vi "Frame.vi"(8 "error in (no error)":errorcluster, 11 "Node Ptr":T1 format="%.0x") -> (0 "error out":errorcluster)   [LabVIEW 2015, in "Diagnostics Addon System Explorer.lvlib"]
uses:
  Diagnostics Addon System Explorer.lvlib
  <vilib>/NI Veristand/Custom Device API/Custom Device Item Ref.ctl
  Shared/FG Action.ctl
  Shared/Signal Parameters FG.vi
  Shared/GUID Lookup.vi
  <vilib>/NI Veristand/Custom Device API/NI VeriStand - Set Item Property.vi
  <vilib>/NI Veristand/Custom Device API/Set Item Property (U32).vi
  <vilib>/NI Veristand/Custom Device API/NI VeriStand - Get Item Property.vi
  <vilib>/NI Veristand/Custom Device API/Get Item Property (U32).vi
  <vilib>/NI Veristand/Custom Device API/NI VeriStand - Get Item Children.vi
  <vilib>/NI Veristand/Custom Device API/Set Item Property (Double).vi
  <vilib>/NI Veristand/Custom Device API/Set Item Property (String).vi
  <vilib>/NI Veristand/Custom Device API/Get Item Property (Double).vi
  <vilib>/NI Veristand/Custom Device API/Get Item Property (String).vi
  <vilib>/NI Veristand/Custom Device API/NI VeriStand - Get Custom Device Channel Data.vi
  <vilib>/NI Veristand/Custom Device API/Custom Device API.lvlib
  Shared/Diagnostics Addon Shared.lvlib
panel:
  out "Length":u32 caption="Length (bytes)"
  in  "ID":u16 format="%.0x"
  out "Signals":i32(listbox)
  in  "Description":string
  in  "Name":string
  in  "SHDocVw.IWebBrowser":refnum<k7>(container)
  in  "Header":cluster{"Section Name":string}={"Section Name"="Custom Device Item Settings"}
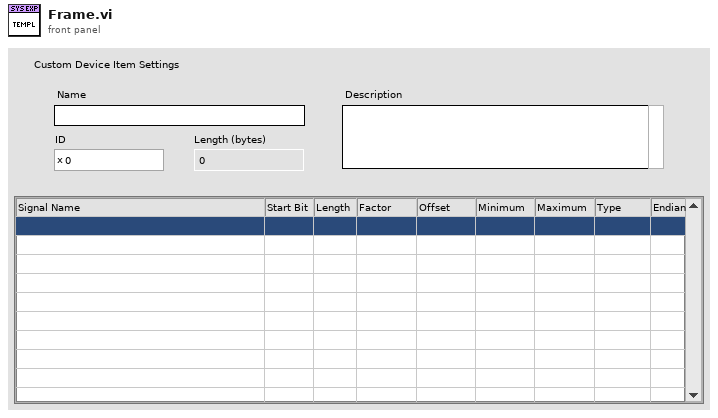
[diagram p1: front panel]
types:
  T1 = typedef "Custom Device API.lvlib/Custom Device Item Ref.ctl" = u64
  T2 = typedef "Diagnostics Addon System Explorer.lvlib/FG Action.ctl" = enum16{"Get", "Set"}
  T3 = typedef "Custom Device API.lvlib/Custom Device Item Info.ctl" = cluster{"Name":string, "Is Channel":bool, "GUID":string, "Is Waveform":bool}
  T4 = typedef "Diagnostics Addon Shared.lvlib/Signal Parameters.ctl" = cluster{"Start Bit":u8, "Length":u8, "Scaling Factor":dbl, "Scaling Offset":dbl, "Minimum":dbl, "Maximum":dbl, "Data Type":u32, "Byte Order":u32, "Default Value":dbl, "Name":string, "Units":string, "Description":string}
  T5 = typedef "Custom Device API.lvlib/Custom Device Commands.ctl" = enum16{"Default", "Item renamed", "Shutdown", "Dynamic button pressed"}
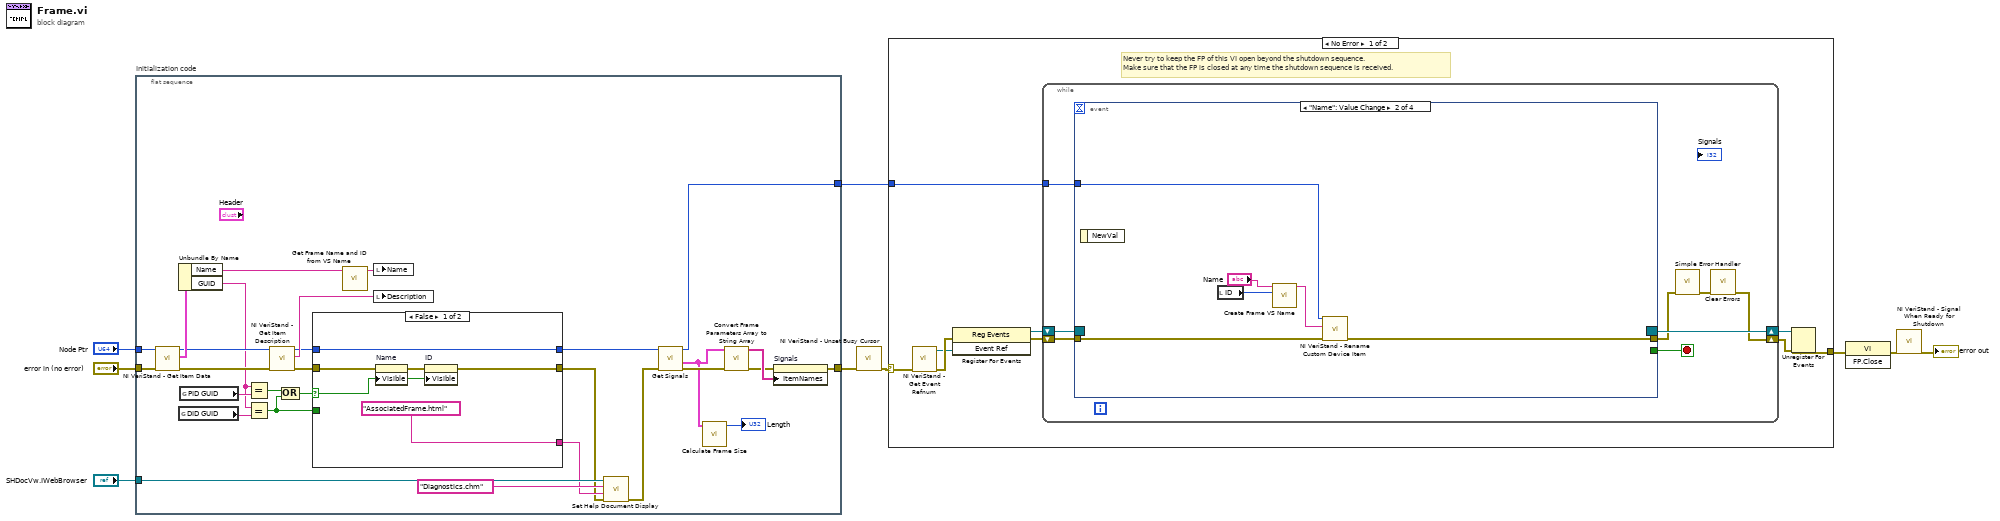
[diagram p0: block diagram]
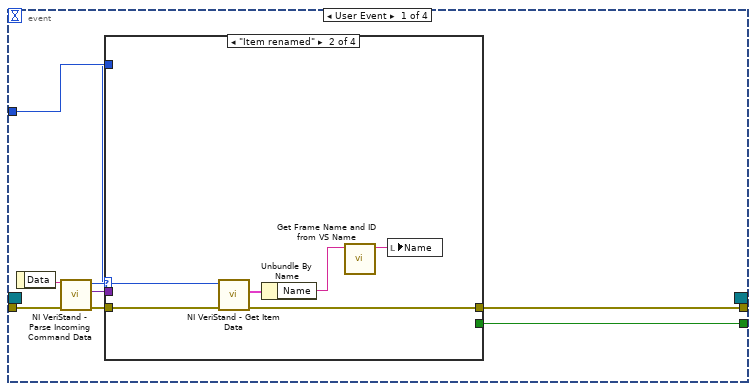
[diagram p2: hidden frame]
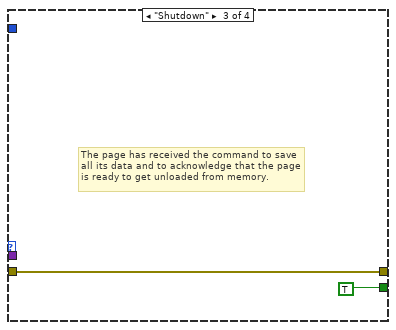
[diagram p4: hidden frame]
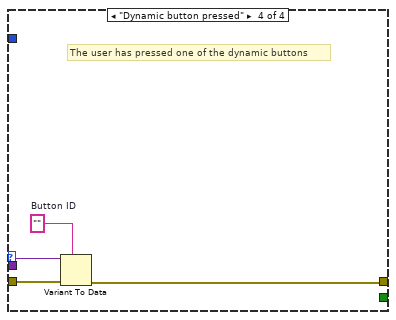
[diagram p5: hidden frame]
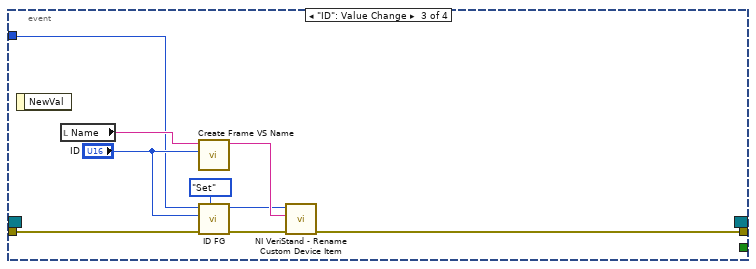
[diagram p6: hidden frame]
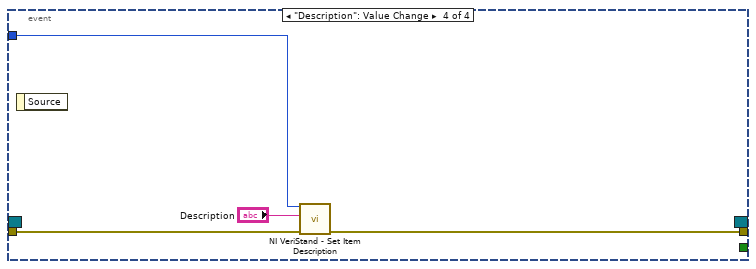
[diagram p7: hidden frame]
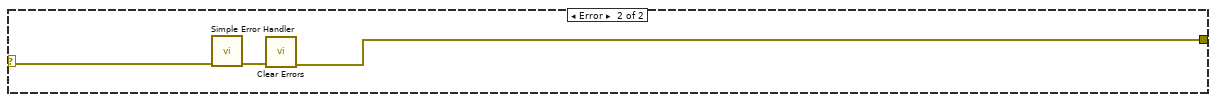
[diagram p8: hidden frame]
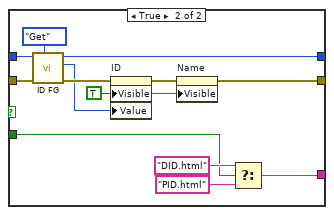
[diagram p9: hidden frame]
diagram:
  n1 = flat-sequence "Initialization code" {
    tunnel: "error in (no error)" -> [w21]
    tunnel: "Node Ptr" -> [w20]
    tunnel: [w33] -> w5
    tunnel: [w36] -> w2
    tunnel: "SHDocVw.IWebBrowser" -> [w19]
    frame #0 {
      n2 = call <vilib>:"NI VeriStand - Get Item Data.vi"("error in (no error)"=w21, "Item Ref in"=w20) -> ("error out"=w22:errorcluster, "Item Info"=w37:T3, "Item Ref out"=w23:T1)  [unwired: 7 out]
      n3 = Unbundle By Name(w37) -> ("Name"=w29:string, "GUID"=w13:string)
      n4 = global read "GUID Lookup.vi" "DID GUID"() -> (w15:string)
      n5 = global read "GUID Lookup.vi" "PID GUID"() -> (w25:string)
      n6 = Equal?(x=w13, y=w25) -> (x = y?=w24:bool)
      n7 = Equal?(x=w13, y=w15) -> (x = y?=w12:bool)
      n8 = call <vilib>:"NI VeriStand - Get Item Description.vi"("error in (no error)"=w22, "Item Ref in"=w23) -> ("error out"=w27:errorcluster, "Description"=w38:string, "Item Ref out"=w26:T1)  [unwired: 7 out]
      n9 = Compound Arithmetic op=OR(w24, w12) -> (w14:bool)
      n10 = case shown="False" w14 {
        selector: w14 -> [w41 _]
        tunnel: [w43 w50] -> w17
        tunnel: [w40 w57] -> w34
        tunnel: w27 -> [w42 w55]
        tunnel: w26 -> [w40 w54]
        tunnel: ["AssociatedFrame.html" ("HTML File") w47] -> w18
        tunnel: w12 -> [_ w45]
        frame False {
          n11 = property on="Name" class="Str"(error in=w42, "Visible"=w41) -> (error out=w44:errorcluster)  [unwired: 1 in, 1 out]
          n12 = property on="ID" class="DigNum (strict)"(error in=w44, "Visible"=w41) -> (error out=w43:errorcluster)  [unwired: 1 in, 1 out]
        }
        frame True {
          w49 = TRUE ("Visible")
          n13 = call "ID FG.vi"("Action"=FG_Action."Get", "error in (no error)"=w55, "Device Item Ref in"=w54) -> ("error out"=w53:errorcluster, "ID"=w52:u32, "Device Item Ref out"=w57:T1)  [unwired: 6 in]
          n14 = property on="ID" class="DigNum (strict)"(error in=w53, "Visible"=w49, "Value"=w52) -> (error out=w51:errorcluster)  [unwired: 1 in, 1 out]
          n15 = property on="Name" class="Str"(error in=w51, "Visible"=w49) -> (error out=w50:errorcluster)  [unwired: 1 in, 1 out]
          n16 = Select(t="DID.html" ("HTML File"), s=w45, f="PID.html" ("HTML File")) -> (s? t:f=w47:string)
        }
      }
      n17 = call "Get Frame Name and ID from VS Name.vi"("VS PID Name"=w29) -> ("PID Name"=w28:string)  [unwired: 9 in, 1 out]
      n18 = local write "Name"(w28) -> ()
      n19 = local write "Description"(w38) -> ()
      n20 = call "Set Help Document Display.vi"("error in (no error)"=w17, "HTML File"=w18, "Main CHM File"="Diagnostics.chm", "SHDocVw.IWebBrowser2"=w19) -> ("error out"=w16:errorcluster)  [unwired: 7 in]
      n21 = call "Get Signals.vi"("error in (no error)"=w16, "Device Item Ref out"=w34) -> ("error out"=w31:errorcluster, "Parameters"=w11:T4[], "Item Ref out"=w36:T1)  [unwired: 6 in, 1 out]
      n22 = call "Calculate Frame Size.vi"("Parameters"=w11) -> ("Bytes"=→"Length":u8)  [unwired: 10 in]
      n23 = call "Convert Frame Parameters Array to String Array.vi"("error in (no error)"=w31, "Frame Parameters"=w11) -> ("error out"=w30:errorcluster, "Frame Parameters"=w32:string[][])  [unwired: 8 in]
      n24 = property on="Signals" class="MCListbox (strict)"(error in=w30, "ItemNames"=w32) -> (error out=w33:errorcluster)  [unwired: 1 in, 1 out]
    }
  }
  n25 = call <vilib>:"NI VeriStand - Unset Busy Cursor.vi"("error in (no error)"=w5) -> ("error out"=w4:errorcluster)  [unwired: 10 out]
  n26 = case shown="No Error" w4 {
    selector: w4 -> [w58 w117]
    tunnel: [w63 w115] -> w9
    tunnel: w2 -> [w59 _]
    frame No Error {
      # "Never try to keep the FP of this VI open beyond the shutdown sequence.\nMake sure that the FP is closed at any time the shutdown sequence is received."
      n27 = call <vilib>:"NI VeriStand - Get Event Refnum.vi"("error in (no error)"=w58) -> ("error out"=w66:errorcluster, "Event Ref"=w62:refnum<user-event>)  [unwired: 9 out]
      n28 = register-events(error in=w66, w62) -> (reference out=w60:refnum<event-registration>, error out=w61:errorcluster)  [unwired: 1 in]
      n29 = while {
        tunnel: w59 -> [w70]
        shift-right: [w67] -> w64
        shift-left: w61 -> [w73]
        shift-right: [w74] -> w65
        shift-left: w60 -> [w72]
        stop <- w71 stop-if-true
        n30 = event shown="[1] \"Name\": Value Change" {
          selector: w72 -> [_ _ _ _]
          dyn-events: [_ _ _ _] -> w74
          timeout: _ -> [_ _ _ _]
          tunnel: w73 -> [w82 w101 w107 w113]
          tunnel: [w78 _ _ _] -> w71
          tunnel: [w77 w100 w109 w112] -> w69
          tunnel: w70 -> [w76 w99 w104 w114]
          event User Event {
            n31 = event-data() -> ("Data"=w81:string)  [unwired: 1 out]
            n32 = call <vilib>:"NI VeriStand - Parse Incoming Command Data.vi"("error in (no error)"=w82, "Incoming data"=w81) -> ("error out"=w80:errorcluster, "Outgoing data"=w75:variant, "Action"=w79:T5)  [unwired: 7 out]
            n33 = case shown="\"Item renamed\"" w79 {
              tunnel: w80 -> [w83 w89 w90 w95]
              tunnel: [_ _ TRUE _] -> w78
              tunnel: [w83 w86 w90 w92] -> w77
              tunnel: w76 -> [_ w88 _ _]
              tunnel: w75 -> [_ _ _ w94]
              frame "Default", Default {
              }
              frame "Item renamed" {
                n34 = call <vilib>:"NI VeriStand - Get Item Data.vi"("error in (no error)"=w89, "Item Ref in"=w88) -> ("error out"=w86:errorcluster, "Item Info"=w87:T3)  [unwired: 8 out]
                n35 = Unbundle By Name(w87) -> ("Name"=w85:string)
                n36 = call "Get Frame Name and ID from VS Name.vi"("VS PID Name"=w85) -> ("PID Name"=w84:string)  [unwired: 9 in, 1 out]
                n37 = local write "Name"(w84) -> ()
              }
              frame "Shutdown" {
                # "The page has received the command to save all its data and to acknowledge that the page is ready to get unloaded from memory."
              }
              frame "Dynamic button pressed" {
                w93 = ""  # Button ID
                # "The user has pressed one of the dynamic buttons"
                n38 = Variant To Data(error in=w95, type=w93, Variant=w94) -> (error out=w92:errorcluster)  [unwired: 1 out]
              }
            }
          }
          event "Name": Value Change {
            n39 = event-data() -> ()  [unwired: 2 out]
            n40 = local read "ID"() -> (w98:u16)
            n41 = call "Create Frame VS Name.vi"("PID Number"=w98, "PID Name"="Name") -> ("VS Name"=w96:string)  [unwired: 9 in]
            n42 = call <vilib>:"NI VeriStand - Rename Custom Device Item.vi"("error in (no error)"=w101, "New Name"=w96, "Item Ref in"=w99) -> ("error out"=w100:errorcluster)  [unwired: 1 in, 7 out]
          }
          event "ID": Value Change {
            n43 = event-data() -> ()  [unwired: 2 out]
            n44 = local read "Name"() -> (w108:string)
            n45 = call "Create Frame VS Name.vi"("PID Number"="ID", "PID Name"=w108) -> ("VS Name"=w110:string)  [unwired: 9 in]
            n46 = call "ID FG.vi"("Action"=FG_Action."Set", "error in (no error)"=w107, "ID"="ID", "Device Item Ref in"=w104) -> ("error out"=w106:errorcluster, "Device Item Ref out"=w103:T1)  [unwired: 5 in, 1 out]
            n47 = call <vilib>:"NI VeriStand - Rename Custom Device Item.vi"("error in (no error)"=w106, "New Name"=w110, "Item Ref in"=w103) -> ("error out"=w109:errorcluster)  [unwired: 1 in, 7 out]
          }
          event "Description": Value Change {
            n48 = event-data() -> ()  [unwired: 2 out]
            n49 = call <vilib>:"NI VeriStand - Set Item Description.vi"("error in (no error)"=w113, "Description"="Description", "Item Ref in"=w114) -> ("error out"=w112:errorcluster)  [unwired: 8 out]
          }
        }
        n50 = call <vilib>:"Simple Error Handler.vi"("error in (no error)"=w69) -> ("error out"=w68:errorcluster)  [unwired: 1 in, 7 out]
        n51 = call <vilib>:"Clear Errors.vi"("error in (no error)"=w68) -> ("error out"=w67:errorcluster)  [unwired: 1 in, 5 out]
      }
      n52 = Unregister For Events(event registration refnum=w65, error in=w64) -> (error out=w63:errorcluster)
    }
    frame Error {
      n53 = call <vilib>:"Simple Error Handler.vi"("error in (no error)"=w117) -> ("error out"=w116:errorcluster)  [unwired: 1 in, 7 out]
      n54 = call <vilib>:"Clear Errors.vi"("error in (no error)"=w116) -> ("error out"=w115:errorcluster)  [unwired: 1 in, 5 out]
    }
  }
  n55 = invoke class="VI" method="FP.Close"(error in=w9) -> (error out=w8:errorcluster)  [unwired: 2 in, 2 out]
  n56 = call <vilib>:"NI VeriStand - Signal When Ready for Shutdown.vi"("error in (no error)"=w8) -> ("error out"=→"error out":errorcluster)  [unwired: 10 out]
